vi "WPI_AnalogTriggerCache.vi"(8 "error in (no error)":errorcluster, 10 "AnalogTriggerToRelease":T1, 11 "Operation":enum16{"Acquire", "Release"}(ring)) -> (0 "error out":errorcluster, 2 "AnalogTriggerAllocated":T1, 3 "Allocated":bool)   [LabVIEW 2017]
doc: "This software is licensed. Open the labview\\readme\\WPI Robotics Library Open Source License.txt file for more information."
uses:
  <vilib>/Rock Robotics/SystemInterfaces/AnalogTrigger/FPGA_AnalogTriggerIndex.ctl
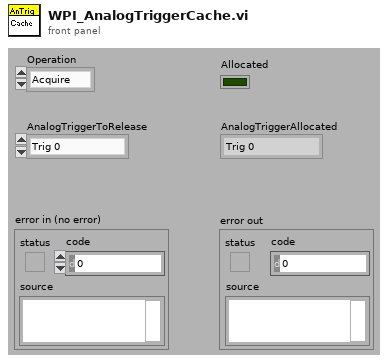
[diagram p1: front panel]
types:
  T1 = typedef "FPGA_AnalogTriggerIndex.ctl" = enum8{"Trig 0", "Trig 1", "Trig 2", "Trig 3", "Trig 4", "Trig 5", "Trig 6", "Trig 7", "Invalid"}
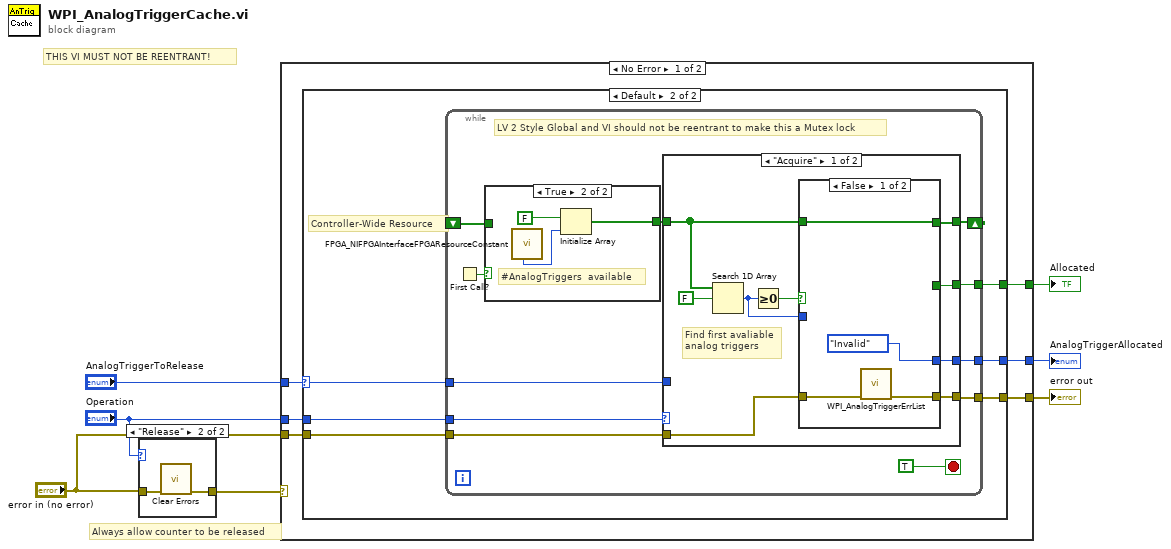
[diagram p0: block diagram]
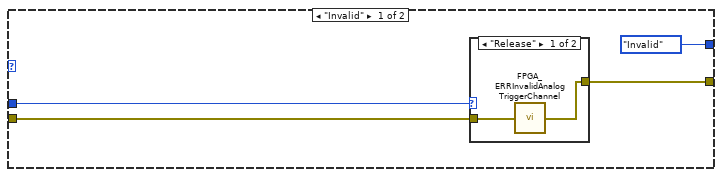
[diagram p3: hidden frame]
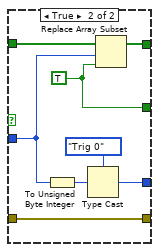
[diagram p5: hidden frame]
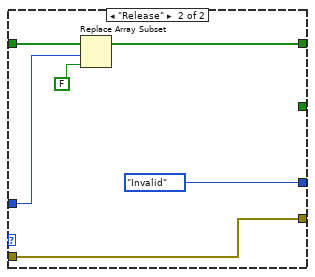
[diagram p6: hidden frame]
diagram:
  # "THIS VI MUST NOT BE REENTRANT!"
  # "Always allow counter to be released"
  n1 = case shown="\"Release\"" "Operation" {
    tunnel: "error in (no error)" -> [w8 w10]
    tunnel: [w8 w9] -> w5
    frame "Acquire", Default {
    }
    frame "Release" {
      n2 = call <vilib>:"Clear Errors.vi"("error in (no error)"=w10) -> ("error out"=w9:errorcluster)  [unwired: 1 in, 5 out]
    }
  }
  n3 = case shown="No Error" w5 {
    selector: w5 -> [_ w72]
    tunnel: "Operation" -> [w16 _]
    tunnel: [w15 w72] -> w1
    tunnel: [w14 _] -> w7
    tunnel: "AnalogTriggerToRelease" -> [w12 _]
    tunnel: [w13 _] -> w3
    tunnel: "error in (no error)" -> [w11 _]
    frame No Error {
      n4 = case shown="Default" w12 {
        selector: w12 -> [_ w25]
        tunnel: w16 -> [w20 w29]
        tunnel: [w19 w28] -> w15
        tunnel: [_ w27] -> w14
        tunnel: [FPGA_AnalogTriggerIndex."Invalid" ("AnalogTriggerAllocated") w26] -> w13
        tunnel: w11 -> [w17 w24]
        frame "Invalid" {
          n5 = case shown="\"Release\"" w20 {
            tunnel: [w22 w23] -> w19
            tunnel: w17 -> [w21 w23]
            frame "Release" {
              n6 = call <vilib>:"FPGA_ERRInvalidAnalogTriggerChannel.vi"("error in (no error)"=w21) -> ("error out"=w22:errorcluster)
            }
            frame "Acquire" {
            }
          }
        }
        frame Default {
          # "Controller-Wide Resource"
          n7 = while {
            shift-right: [w37] -> _
            shift-left: _ -> [w39]
            tunnel: w29 -> [w38]
            tunnel: w25 -> [w33]
            tunnel: [w36] -> w28
            tunnel: [w35] -> w27
            tunnel: [w32] -> w26
            tunnel: w24 -> [w30]
            stop <- TRUE stop-if-true
            # "LV 2 Style Global and VI should not be reentrant to make this a Mutex lock"
            n8 = First Call?() -> (First Call?: T/F=w40:bool)
            n9 = case shown="True" w40 {
              tunnel: w39 -> [w68 _]
              tunnel: [w68 w70] -> w34
              frame False {
              }
              frame True {
                # "#AnalogTriggers  available"
                n10 = call <vilib>:"FPGA_NIFPGAInterfaceFPGAResourceConstant.vi"() -> ("NumberOfAnalogTriggers"=w69:u32)  [unwired: 11 out]
                n11 = Initialize Array(FALSE, w69) -> (w70:bool[])
              }
            }
            n12 = case shown="\"Acquire\"" w38 {
              tunnel: w34 -> [w45 w67]
              tunnel: [w49 w66] -> w37
              tunnel: w33 -> [_ w65]
              tunnel: [w48 w62] -> w36
              tunnel: [w47 _] -> w35
              tunnel: [w46 FPGA_AnalogTriggerIndex."Invalid" ("AnalogTriggerAllocated")] -> w32
              tunnel: w30 -> [w41 w62]
              frame "Acquire" {
                # "Find first avaliable\nanalog triggers"
                n13 = Search 1D Array(1D array=w45, element=FALSE) -> (index of element=w42:i32)  [unwired: 1 out]
                n14 = Greater Or Equal To 0?(x=w42) -> (x >= 0?=w43:bool)
                n15 = case shown="False" w43 {
                  tunnel: w45 -> [w53 w60]
                  tunnel: [w53 w59] -> w49
                  tunnel: w42 -> [_ w58]
                  tunnel: [w50 w54] -> w48
                  tunnel: [_ w61] -> w47
                  tunnel: [FPGA_AnalogTriggerIndex."Invalid" ("AnalogTriggerAllocated") w57] -> w46
                  tunnel: w41 -> [w51 w54]
                  frame False {
                    n16 = call <vilib>:"WPI_AnalogTriggerErrList.vi"("error in (no error)"=w51) -> ("error out"=w50:errorcluster)  [unwired: 2 in, 8 out]
                  }
                  frame True {
                    w61 = TRUE ("new element/subarray")
                    n17 = To Unsigned Byte Integer(number=w58) -> (unsigned 8bit integer=w55:u8)
                    n18 = Type Cast(type=FPGA_AnalogTriggerIndex."Trig 0" ("AnalogTriggerAllocated"), x=w55) -> (*(type *) &x=w57:T1)
                    n19 = Replace Array Subset(array=w60, new element=w61, index=w58) -> (w59:bool[])
                  }
                }
              }
              frame "Release" {
                n20 = Replace Array Subset(array=w67, new element=FALSE ("new element/subarray"), index=w65) -> (w66:bool[])
              }
            }
          }
        }
      }
    }
    frame Error {
    }
  }
  "Allocated" <- w7
  "error out" <- w1
  "AnalogTriggerAllocated" <- w3
